vi "Parse Text-& UnescapedVariable-Text.vi"(8 "Error In":errorcluster) -> (0 "Error Out":errorcluster)   [LabVIEW 2018, in "Tests.lvlib" / "Parser.lvlib"]
uses:
  Parser.lvlib
  src/Toolkit/Public/Tokens/Text/Text.lvclass
  src/Toolkit/Public/Tokens/UnescapedVariable/UnescapedVariable.lvclass
  src/Toolkit/Public/Readers/Public/String/String.lvclass
  D:/Users/cfield/Code/Field R&D Services/Mustache/trunk/src/Mustache/Public/Readers/Public/Abstract/Abstract.lvclass
  <vilib>/Utility/LVClass/Get LV Class Name.vi
  src/Toolkit/Public/Tokens/Text/API/Read Content.vi
  <vilib>/addons/_JKI Toolkits/Caraya/classes/Assert/Assert Equal_Variant.vi
  src/Toolkit/Public/Tokens/Keyable/API/Keyable.lvclass
  <vilib>/addons/_JKI Toolkits/Caraya/classes/Test/Test.lvclass
  src/Toolkit/Public/Parser/Parser.lvclass
  <vilib>/addons/_JKI Toolkits/Caraya/classes/Assert/Assert.lvclass
  src/Toolkit/Public/Tokens/Abstract/Abstract.lvclass
  Tests.lvlib
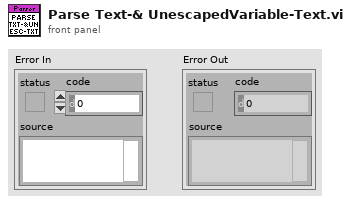
[diagram p1: front panel]
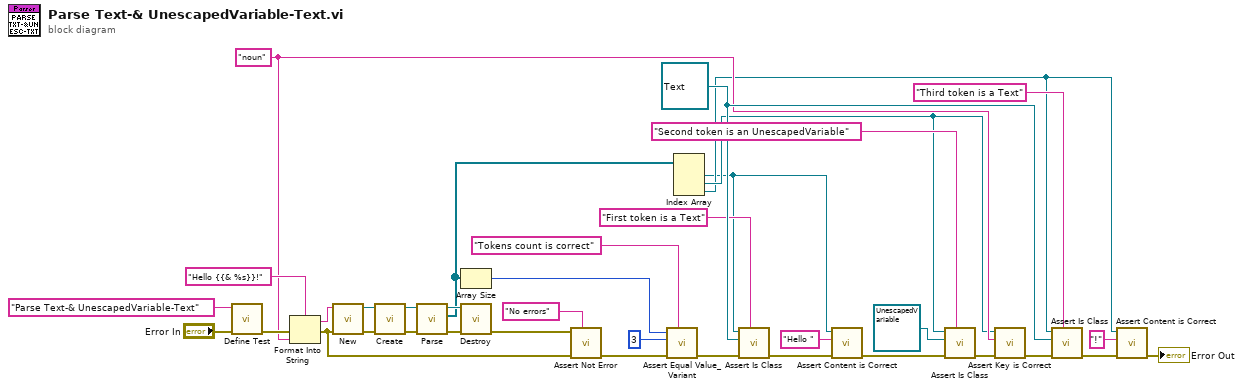
[diagram p0: block diagram]
diagram:
  w11 = refnum<class "Text.lvclass"> refnum ("Mustache.lvlib:Tokens.lvlib:Text.lvclass")
  w7 = "noun" ("String")
  n1 = call <vilib>:"Define Test.vi"("error in (no error)"="Error In", "Label (VI Title)"="Parse Text-& UnescapedVariable-Text") -> ("error out"=w28:errorcluster)  [unwired: 9 in]
  n2 = Format Into String(format string="Hello {{& %s}}!", error in=w28, w7) -> (resulting string=w18:string, error out=w20:errorcluster)  [unwired: 1 in]
  n3 = call "New.vi"("Error In"=w20, "String"=w18) -> ("Error Out"=w34:errorcluster, "String"=w35:refnum<class "String.lvclass">)  [unwired: 8 in]
  n4 = call "Create.vi"("Error In"=w34, "Reader"=w35) -> ("Error Out"=w33:errorcluster, "Parser"=w32:refnum<class "Parser.lvclass">)  [unwired: 8 in]
  n5 = call "Parse.vi"("Error In"=w33, "Parser In"=w32) -> ("Error Out"=w30:errorcluster, "Tokens"=w21:refnum<class "Abstract.lvclass">[], "Parser Out"=w31:refnum<class "Parser.lvclass">)  [unwired: 7 in]
  n6 = Array Size(array=w21) -> (size(s)=w24:i32)
  n7 = call "Destroy.vi"("Error In"=w30, "Parser"=w31) -> ("Error Out"=w29:errorcluster)  [unwired: 9 in]
  n8 = call <vilib>:"Assert Not Error.vi"("Label"="No errors", "error in (no error)"=w20, "Not Error?"=w29) -> ("error out"=w26:errorcluster)  [unwired: 8 in]
  n9 = call <vilib>:"Assert Equal Value_Variant.vi"("Label"="Tokens count is correct", "error in (no error)"=w26, "Y"=3 ("size(s)"), "X"=w24) -> ("error out"=w22:errorcluster)  [unwired: 7 in]
  n10 = Index Array(array=w21) -> (element #1=w1:refnum<class "Abstract.lvclass">, element #2=w5:refnum<class "Abstract.lvclass">, element #3=w3:refnum<class "Abstract.lvclass">)  [unwired: 3 in]
  n11 = call "Assert Is Class.vi"("Label"="First token is a Text", "Error In"=w22, "Expected"=w11, "Actual"=w1) -> ("Error Out"=w17:errorcluster)  [unwired: 7 in]
  n12 = call "Assert Content is Correct.vi"("Error In"=w17, "Expected"="Hello ", "Token"=w1) -> ("Error Out"=w16:errorcluster)  [unwired: 8 in]
  n13 = call "Assert Is Class.vi"("Label"="Second token is an UnescapedVariable", "Error In"=w16, "Expected"=refnum<class "UnescapedVariable.lvclass"> refnum ("Mustache.lvlib:Tokens.lvlib:UnescapedVariable.lvclass"), "Actual"=w5) -> ("Error Out"=w6:errorcluster)  [unwired: 7 in]
  n14 = call "Assert Key is Correct.vi"("Error In"=w6, "Expected"=w7, "Token"=w5) -> ("Error Out"=w15:errorcluster)  [unwired: 8 in]
  n15 = call "Assert Is Class.vi"("Label"="Third token is a Text", "Error In"=w15, "Expected"=w11, "Actual"=w3) -> ("Error Out"=w14:errorcluster)  [unwired: 7 in]
  n16 = call "Assert Content is Correct.vi"("Error In"=w14, "Expected"="!", "Token"=w3) -> ("Error Out"=→"Error Out":errorcluster)  [unwired: 8 in]
